vi "Create Sysdef Tree from DB Channel Clusters_RTs_Create SAs.vi"(5 "messageBuffers":T3(array[cluster]), 6 "Autocreate Rx timestamp chans?":bool, 7 "subAddresses":T4[](array[typedef]), 8 "error in (no error)":errorcluster, 10 "rtMode":T1, 11 "Section Ptr in":T2 format="%.0x") -> (0 "error out":errorcluster, 3 "Section Ptr out":T2 format="%.0x")   [LabVIEW 2020, in "Ballard 1553 System Explorer.lvlib"]
uses:
  Ballard 1553 System Explorer.lvlib
  <vilib>/NI VeriStand/Custom Device API/Custom Device Item Ref.ctl
  Parse XML Ballard/Ballard_RT subAddress.ctl
  Parse XML Ballard/Ballard_RT direction.ctl
  Parse XML Ballard/Ballard_RT rtMode.ctl
  <vilib>/NI VeriStand/Custom Device API/Custom Device Channel.ctl
  <vilib>/NI VeriStand/Custom Device API/Custom Device Channel Type.ctl
  Shared/Controls and Global/Global.vi
  <vilib>/NI VeriStand/Custom Device API/Set Item Property (I32).vi
  <vilib>/NI VeriStand/Custom Device API/Set Item Property (U16).vi
  <userlib>/_OpenG.lib/array/array.llb/Remove Duplicates from 1D Array (I8)__ogtk.vi
  <vilib>/NI VeriStand/Custom Device API/Custom Device API.lvlib
  Shared/Ballard 1553 Shared.lvlib
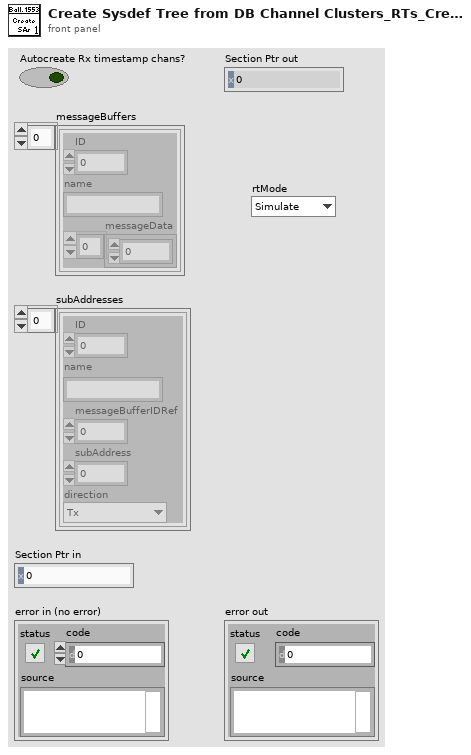
[diagram p1: front panel]
types:
  T1 = typedef "Ballard 1553 System Explorer.lvlib/Ballard_RT rtMode.ctl" = enum16{"Simulate", "Monitor", "Disable"}
  T2 = typedef "Custom Device API.lvlib/Custom Device Item Ref.ctl" = u64
  T3 = cluster{"ID":i32, "name":string, "messageData":u16[]}[]
  T4 = typedef "Ballard 1553 System Explorer.lvlib/Ballard_RT subAddress.ctl" = cluster{"ID":i32, "name":string, "messageBufferIDRef":i32, "subAddress":i8, "direction":T5}
  T5 = typedef "Ballard 1553 System Explorer.lvlib/Ballard_RT direction.ctl" = enum16{"Tx", "Rx"}
  T6 = typedef "Custom Device API.lvlib/Custom Device Channel Type.ctl" = enum16{"Input", "Output"}
  T7 = typedef "Custom Device API.lvlib/Custom Device Channel.ctl" = cluster{"Type":T6, "Units":string, "Default Value":dbl, "Faultable":bool, "Scalable":bool}
  T8 = enum16{"DW", "STC", "SPC", "SW", "TI MC", "AC", "TI WC"}
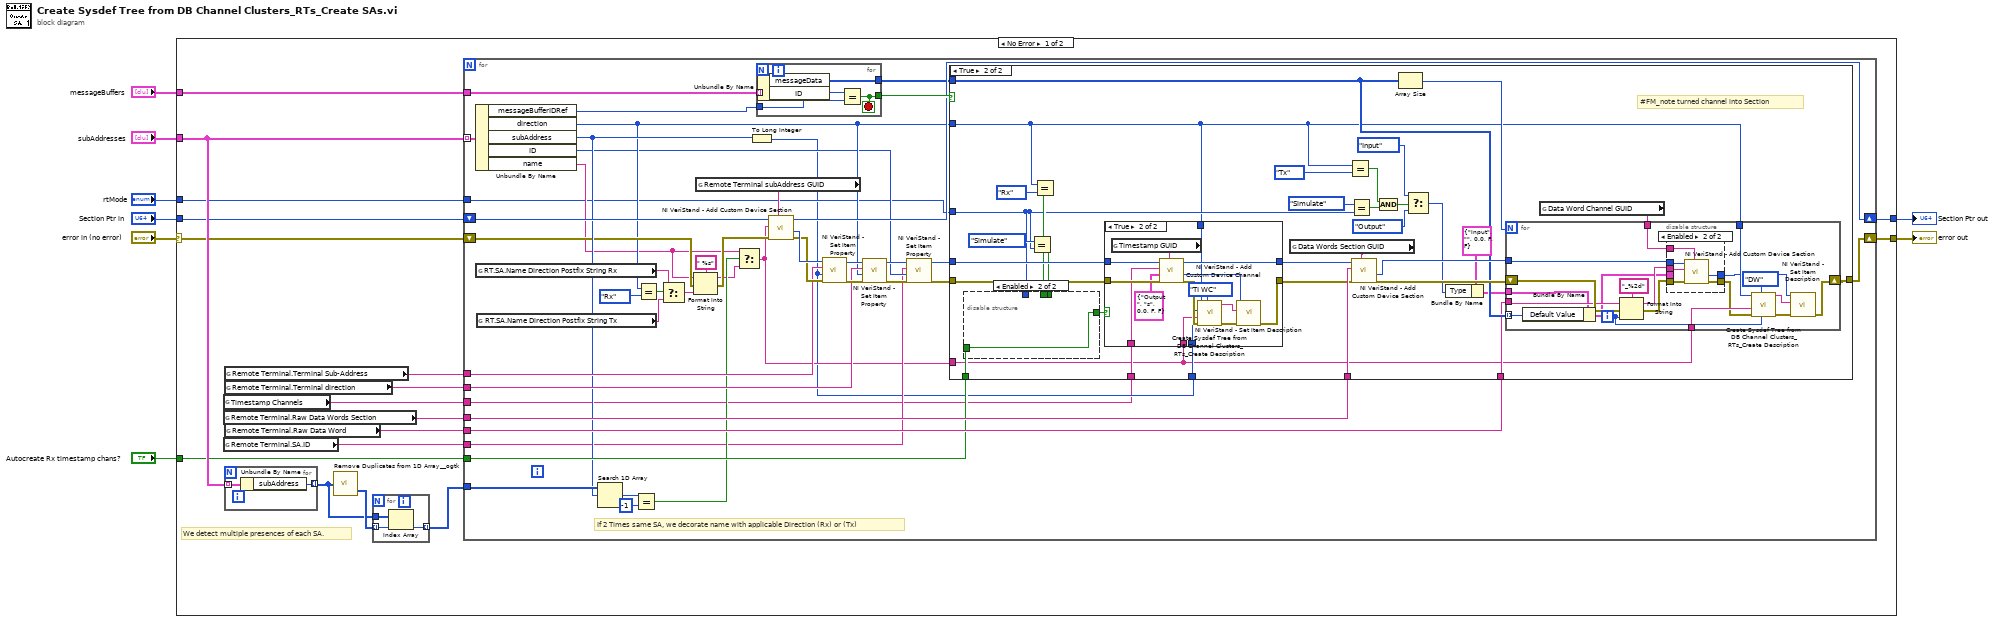
[diagram p0: block diagram]
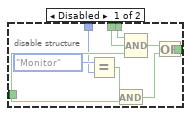
[diagram p3: hidden frame]
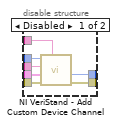
[diagram p5: hidden frame]
diagram:
  n1 = case shown="No Error" "error in (no error)" {
    selector: "error in (no error)" -> [w10 w175]
    tunnel: [w25 w174] -> w8
    tunnel: [w24 w175] -> w7
    tunnel: "subAddresses" -> [w19 _]
    tunnel: "Autocreate Rx timestamp chans?" -> [w17 _]
    tunnel: "messageBuffers" -> [w16 _]
    tunnel: "Section Ptr in" -> [w13 w174]
    tunnel: "rtMode" -> [w9 _]
    frame No Error {
      # "We detect multiple presences of each SA."
      n2 = global read "Global.vi" "Timestamp Channels"() -> (w18:string)
      n3 = global read "Global.vi" "Remote Terminal.Raw Data Words Section"() -> (w14:string)
      n4 = global read "Global.vi" "Remote Terminal.SA.ID"() -> (w23:string)
      n5 = global read "Global.vi" "Remote Terminal.Terminal Sub-Address"() -> (w11:string)
      n6 = global read "Global.vi" "Remote Terminal.Terminal direction"() -> (w12:string)
      n7 = global read "Global.vi" "Remote Terminal.Raw Data Word"() -> (w15:string)
      n8 = for {
        tunnel: w19 -> [w30] mode=indexing
        tunnel: [w29] -> w20 mode=indexing
        n9 = Unbundle By Name(w30) -> ("subAddress"=w29:i8)
      }
      n10 = call-poly <userlib>:"Remove Duplicates from 1D Array__ogtk.vi"("Input Array"=w20) -> ("indices of removed elements"=w21:i32[])  [unwired: 1 out]
      n11 = for {
        tunnel: w20 -> [w27]
        tunnel: w21 -> [w28] mode=indexing
        tunnel: [w26] -> w22 mode=indexing
        n12 = Index Array(array=w27, index=w28) -> (element=w26:i8)
      }
      n13 = for {
        tunnel: w19 -> [w74] mode=indexing
        shift-right: [w60] -> w24
        shift-left: w10 -> [w49]
        shift-right: [w61] -> w25
        shift-left: w13 -> [w73]
        tunnel: w11 -> [w70]
        tunnel: w12 -> [w67]
        tunnel: w14 -> [w65]
        tunnel: w15 -> [w58]
        tunnel: w16 -> [w64]
        tunnel: w17 -> [w57]
        tunnel: w18 -> [w31]
        tunnel: w22 -> [w56]
        tunnel: w23 -> [w35]
        tunnel: w9 -> [w34]
        # "If 2 Times same SA, we decorate name with applicable Direction (Rx) or (Tx)"
        n14 = Unbundle By Name(w74) -> ("messageBufferIDRef"=w63:i32, "direction"=w47:T5, "subAddress"=w55:i8, "ID"=w36:i32, "name"=w37:string)
        n15 = global read "Global.vi" "RT.SA.Name Direction Postfix String Rx"() -> (w45:string)
        n16 = global read "Global.vi" "RT.SA.Name Direction Postfix String Tx"() -> (w46:string)
        n17 = Search 1D Array(1D array=w56, element=w55) -> (index of element=w54:i32)  [unwired: 1 in]
        n18 = Equal?(x=w54, y=-1) -> (x = y?=w52:bool)
        n19 = Equal?(x=w47, y=Ballard_RT_direction."Rx") -> (x = y?=w50:bool)
        n20 = Select(t=w45, s=w50, f=w46) -> (s? t:f=w44:string)
        n21 = Format Into String(format string=" %s", initial string=w37, error in=w49, w44) -> (resulting string=w42:string, error out=w48:errorcluster)
        n22 = global read "Global.vi" "Remote Terminal subAddress GUID"() -> (w66:string)
        n23 = Select(t=w37, s=w52, f=w42) -> (s? t:f=w33:string)
        n24 = To Long Integer(number=w55) -> (32bit integer=w32:i32)
        n25 = for {
          tunnel: w64 -> [w173] mode=indexing
          tunnel: w63 -> [w171]
          tunnel: [w170] -> w59
          tunnel: [w169] -> w62
          stop <- w169 stop-if-true
          n26 = Unbundle By Name(w173) -> ("messageData"=w170:u16[], "ID"=w172:i32)
          n27 = Equal?(x=w172, y=w171) -> (x = y?=w169:bool)
        }
        n28 = call <vilib>:"NI VeriStand - Add Custom Device Section.vi"("GUID (Default Section)"=w66, "error in (no error)"=w48, "Section Name"=w33, "Parent Ref in"=w73) -> ("error out"=w71:errorcluster, "Section Ptr"=w72:T2, "Parent Ref out"=w61:T2)  [unwired: 4 in, 1 out]
        n29 = call-poly <vilib>:"NI VeriStand - Set Item Property.vi"("error in (no error)"=w71, "Value"=w32, "Property Name"=w70, "Item Ref in"=w72) -> ("error out"=w69:errorcluster, "Item Ref out"=w68:T2)  [unwired: 5 in, 1 out]
        n30 = call-poly <vilib>:"NI VeriStand - Set Item Property.vi"("error in (no error)"=w69, "Value"=w47, "Property Name"=w67, "Item Ref in"=w68) -> ("error out"=w40:errorcluster, "Item Ref out"=w41:T2)  [unwired: 5 in, 1 out]
        n31 = call-poly <vilib>:"NI VeriStand - Set Item Property.vi"("error in (no error)"=w40, "Value"=w36, "Property Name"=w35, "Item Ref in"=w41) -> ("error out"=w38:errorcluster, "Item Ref out"=w39:T2)  [unwired: 5 in, 1 out]
        n32 = case shown="True" w62 {
          tunnel: w38 -> [w75 w89]
          tunnel: w65 -> [_ w109]
          tunnel: w39 -> [_ w90]
          tunnel: [w75 w92] -> w60
          tunnel: w59 -> [_ w104]
          tunnel: w58 -> [_ w103]
          tunnel: w34 -> [_ w80]
          tunnel: w47 -> [_ w77]
          tunnel: w57 -> [_ w85]
          tunnel: w31 -> [_ w79]
          tunnel: w33 -> [_ w76]
          tunnel: w32 -> [_ w78]
          frame False {
          }
          frame True {
            # "#FM_note turned channel into Section"
            n33 = Equal?(x=Ballard_RT_rtMode."Simulate", y=w80) -> (x = y?=w83:bool)
            n34 = Equal?(x=w77, y=Ballard_RT_direction."Rx") -> (x = y?=w81:bool)
            n35 = disable-structure shown="Enabled" {
              disable-tunnel: [w118 w119] -> w86
              disable-tunnel: w85 -> [w114 w119]
              disable-tunnel: w83 -> [w112 _]
              disable-tunnel: w81 -> [w111 _]
              disable-tunnel: w80 -> [w110 _]
              frame Disabled {
                n36 = Equal?(x=Ballard_RT_rtMode."Monitor", y=w110) -> (x = y?=w116:bool)
                n37 = And(x=w116, y=w114) -> (x .and. y?=w115:bool)
                n38 = Compound Arithmetic op=AND(w112, w111, w114) -> (w113:bool)
                n39 = Or(x=w113, y=w115) -> (x .or. y?=w118:bool)
              }
              frame Enabled {
              }
            }
            n40 = case shown="True" w86 {
              tunnel: w90 -> [w121 w136]
              tunnel: w89 -> [w120 w135]
              tunnel: [w121 w134] -> w88
              tunnel: [w120 w128] -> w87
              tunnel: w79 -> [_ w131]
              tunnel: w76 -> [_ w125]
              tunnel: w78 -> [_ w124]
              tunnel: w77 -> [_ w123]
              frame False {
              }
              frame True {
                n41 = global read "Global.vi" "Timestamp GUID"() -> (w133:string)
                n42 = call <vilib>:"NI VeriStand - Add Custom Device Channel.vi"("GUID (Default Channel)"=w133, "error in (no error)"=w135, "Channel"=T7 {"Type"=enum."Output", "Units"="s", "Default Value"=0.0, "Faultable"=FALSE, "Scalable"=FALSE}, "Channel Name"=w131, "Parent Ref in"=w136) -> ("error out"=w129:errorcluster, "Channel Ref"=w126:T2, "Parent Ref out"=w134:T2)  [unwired: 3 in, 1 out]
                n43 = call "Create Sysdef Tree from DB Channel Clusters_RTs_Create Description.vi"("Type"=T8."TI WC", "error in (no error)"=w129, "Name"=w125, "SA/MC"=w124, "Direction"=w123) -> ("error out"=w130:errorcluster, "Description (Out)"=w127:string)  [unwired: 5 in]
                n44 = call <vilib>:"NI VeriStand - Set Item Description.vi"("error in (no error)"=w130, "Description"=w127, "Item Ref in"=w126) -> ("error out"=w128:errorcluster)  [unwired: 6 in, 2 out]
              }
            }
            n45 = global read "Global.vi" "Data Words Section GUID"() -> (w91:string)
            n46 = Equal?(x=w77, y=Ballard_RT_direction."Tx") -> (x = y?=w97:bool)
            n47 = Equal?(x=Ballard_RT_rtMode."Simulate", y=w80) -> (x = y?=w99:bool)
            n48 = call <vilib>:"NI VeriStand - Add Custom Device Section.vi"("GUID (Default Section)"=w91, "error in (no error)"=w87, "Section Name"=w109, "Parent Ref in"=w88) -> ("error out"=w108:errorcluster, "Section Ptr"=w107:T2)  [unwired: 4 in, 2 out]
            n49 = And(x=w97, y=w99) -> (x .and. y?=w96:bool)
            n50 = Array Size(array=w104) -> (size(s)=w105:i32)
            n51 = Select(t=Custom_Device_Channel_Type."Input" ("Type"), s=w96, f=Custom_Device_Channel_Type."Output") -> (s? t:f=w94:T6)
            n52 = Bundle By Name(cluster=T7 {"Type"=enum."Input", "Units"="", "Default Value"=0.0, "Faultable"=FALSE, "Scalable"=FALSE} ("Channel"), "Type"=w94) -> (w101:T7)
            n53 = global read "Global.vi" "Data Word Channel GUID"() -> (w106:string)
            n54 = for {
              N: w105 -> [_]
              tunnel: w107 -> [w143]
              tunnel: w103 -> [w152]
              shift-right: [w147] -> w92
              shift-left: w108 -> [w154]
              tunnel: w104 -> [w153] mode=indexing
              tunnel: w106 -> [w137]
              tunnel: w101 -> [w151]
              tunnel: w77 -> [w145]
              tunnel: w76 -> [w144]
              i -> [w149]
              n55 = Bundle By Name(cluster=w151, "Default Value"=w153) -> (w141:T7)
              n56 = Format Into String(format string="_%2d", initial string=w152, error in=w154, w149) -> (resulting string=w142:string, error out=w140:errorcluster)
              n57 = disable-structure shown="Enabled" {
                disable-tunnel: w143 -> [w162 w165]
                disable-tunnel: w140 -> [w161 w167]
                disable-tunnel: w142 -> [w160 w163]
                disable-tunnel: w141 -> [w159 _]
                disable-tunnel: w137 -> [w158 w164]
                disable-tunnel: [w157 w166] -> w138
                disable-tunnel: [w156 w168] -> w139
                frame Disabled {
                  n58 = call <vilib>:"NI VeriStand - Add Custom Device Channel.vi"("GUID (Default Channel)"=w158, "error in (no error)"=w161, "Channel"=w159, "Channel Name"=w160, "Parent Ref in"=w162) -> ("error out"=w156:errorcluster, "Channel Ref"=w157:T2)  [unwired: 3 in, 2 out]
                }
                frame Enabled {
                  n59 = call <vilib>:"NI VeriStand - Add Custom Device Section.vi"("GUID (Default Section)"=w164, "error in (no error)"=w167, "Section Name"=w163, "Parent Ref in"=w165) -> ("error out"=w168:errorcluster, "Section Ptr"=w166:T2)  [unwired: 4 in, 2 out]
                }
              }
              n60 = call "Create Sysdef Tree from DB Channel Clusters_RTs_Create Description.vi"("Word Index"=w149, "Type"=T8."DW", "error in (no error)"=w139, "Name"=w144, "Direction"=w145) -> ("error out"=w150:errorcluster, "Description (Out)"=w148:string)  [unwired: 5 in]
              n61 = call <vilib>:"NI VeriStand - Set Item Description.vi"("error in (no error)"=w150, "Description"=w148, "Item Ref in"=w138) -> ("error out"=w147:errorcluster)  [unwired: 6 in, 2 out]
            }
          }
        }
      }
    }
    frame Error {
    }
  }
  "Section Ptr out" <- w8
  "error out" <- w7
